vi "Set Object ACL.vi"(6 "Version ID":string, 8 "error in (no error)":errorcluster, 9 "Access Control Policy":T1, 10 "Object Path":string, 11 "Bucket in":refnum<class "Bucket.lvclass">) -> (0 "error out":errorcluster, 3 "Bucket out":refnum<class "Bucket.lvclass">)   [LabVIEW 2015, in "NI_AWS_S3.lvlib" / "Bucket.lvclass"]
uses:
  Bucket.lvclass
  Access Control Policy.ctl
  User.ctl
  Grantee-Permission Pair.ctl
  Permission.ctl
  Core/HTTP Request/Request Options.ctl
  Core/HTTP Request/Name Value Pair.ctl
  Core/HTTP Request/Region handling.ctl
  Core/HTTP Request/URL formatting.ctl
  Bucket.lvclass/Bucket.ctl
  Read Name.vi
  Core/HTTP Request/HTTP Request.lvclass
  NI_AWS_S3.lvlib
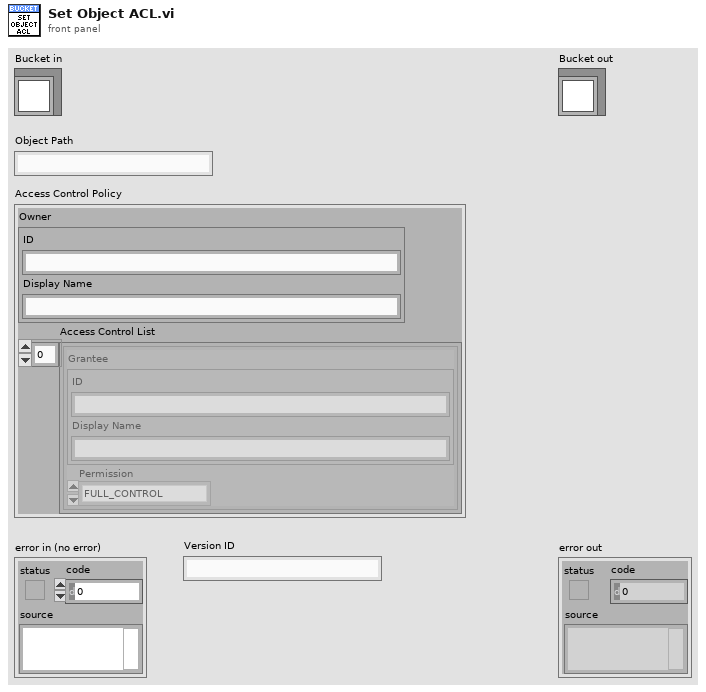
[diagram p1: front panel]
types:
  T1 = typedef "NI_AWS_S3.lvlib/Access Control Policy.ctl" = cluster{"Owner":T2, "Access Control List":T3[]}
  T2 = typedef "NI_AWS_S3.lvlib/User.ctl" = cluster{"ID":string, "Display Name":string}
  T3 = typedef "NI_AWS_S3.lvlib/Grantee-Permission Pair.ctl" = cluster{"Grantee":T2, "Permission":T4}
  T4 = typedef "NI_AWS_S3.lvlib/Permission.ctl" = enum16{"FULL_CONTROL", "WRITE", "WRITE_ACP", "READ", "READ_ACP"}
  T5 = typedef "NI_AWS_Core.lvlib/HTTP Request.lvclass/Name Value Pair.ctl" = cluster{"name":string, "value":string}
  T6 = typedef "NI_AWS_Core.lvlib/HTTP Request.lvclass/Region handling.ctl" = enum16{"use region everywhere", "use region (authentication only)", "use region (URL only)", "ignore region everwhere"}
  T7 = typedef "NI_AWS_Core.lvlib/HTTP Request.lvclass/Request Options.ctl" = cluster{"request headers":T5[], "request parameters":T5[], "request body":string, "region handling":T6, "URL formatting":T8}
  T8 = typedef "NI_AWS_Core.lvlib/HTTP Request.lvclass/URL formatting.ctl" = enum16{"region-", "region."}
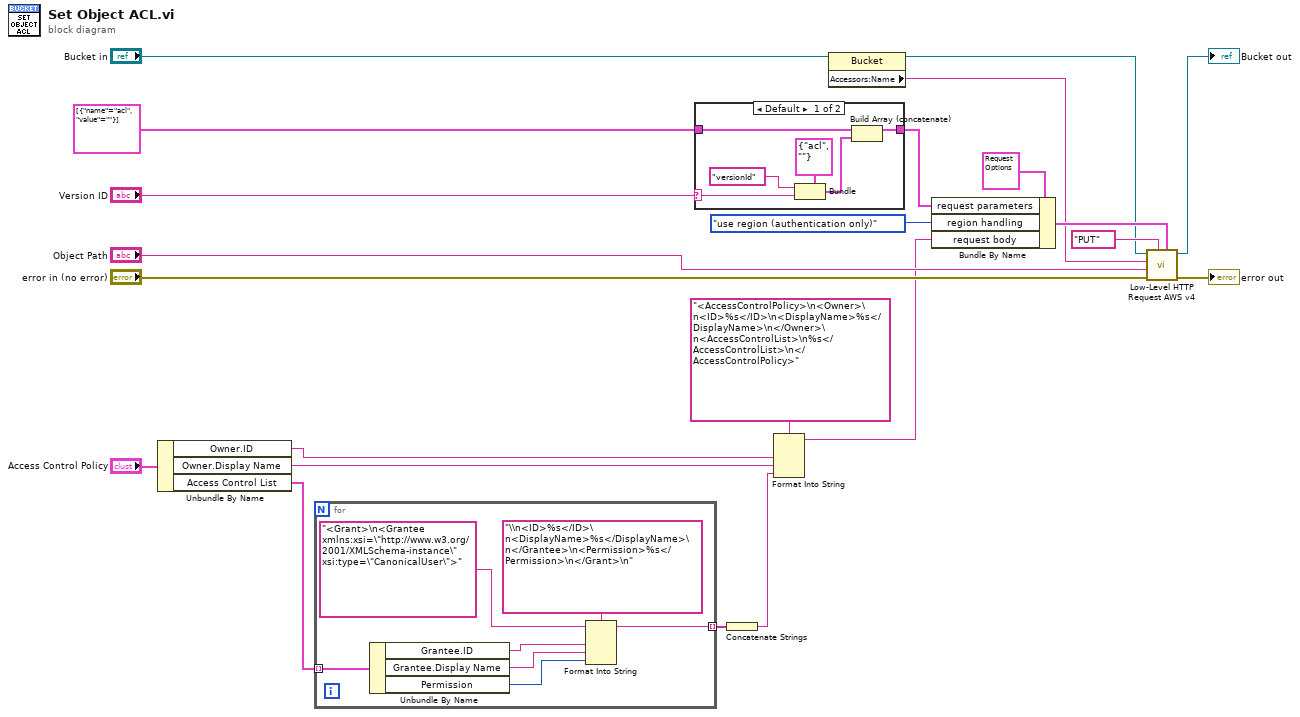
[diagram p0: block diagram]
diagram:
  n1 = Unbundle By Name("Access Control Policy") -> ("Owner.ID"=w5:string, "Owner.Display Name"=w6:string, "Access Control List"=w4:T3[])
  n2 = for {
    tunnel: w4 -> [w29] mode=indexing
    tunnel: [w23] -> w3 mode=indexing
    n3 = Unbundle By Name(w29) -> ("Grantee.ID"=w26:string, "Grantee.Display Name"=w25:string, "Permission"=w24:T4)
    n4 = Format Into String(format string="\\n<ID>%s</ID>\n<DisplayName>%s</DisplayName>\n</Grantee>\n<Permission>%s</Permission>\n</Grant>\n", initial string="<Grant>\n<Grantee xmlns:xsi=\"http://www.w3.org/2001/XMLSchema-instance\" xsi:type=\"CanonicalUser\">", w26, w25, w24) -> (resulting string=w23:string)  [unwired: 1 in, 1 out]
  }
  n5 = case shown="Default" "Version ID" {
    selector: "Version ID" -> [w32 _]
    tunnel: [w33 w36] -> w18
    tunnel: T5[] [{"name"="acl", "value"=""}] ("appended array") -> [w31 w36]
    frame Default {
      n6 = Bundle(cluster=T5 {"name"="acl", "value"=""}, "name"="versionId", "value"=w32) -> (w34:T5)
      n7 = Build Array (concatenate)(w31, w34) -> (w33:T5[])
    }
    frame "" {
    }
  }
  n8 = Concatenate Strings(w3) -> (w2:string)
  n9 = Format Into String(format string="<AccessControlPolicy>\n<Owner>\n<ID>%s</ID>\n<DisplayName>%s</DisplayName>\n</Owner>\n<AccessControlList>\n%s</AccessControlList>\n</AccessControlPolicy>", w5, w6, w2) -> (resulting string=w8:string)  [unwired: 2 in, 1 out]
  n10 = property class="Bucket"(reference="Bucket in") -> (reference out=w14:refnum<class "Bucket.lvclass">, "Accessors:Name"=w13:string)  [unwired: 1 in, 1 out]
  n11 = Bundle By Name(cluster=T7 {"request headers"=[], "request parameters"=[], "request body"="", "region handling"=enum."use region everywhere", "URL formatting"=enum."region."} ("Request Options"), "request parameters"=w18, "region handling"=Region_handling."use region (authentication only)", "request body"=w8) -> (w19:T7)
  n12 = call "Low-Level HTTP Request AWS v4.vi"("Request Options"=w19, "HTTP-Verb"="PUT", "error in (no error)"="error in (no error)", "URL Suffix"="Object Path", "URL Prefix"=w13, "AWS Core in"=w14) -> ("error out"=→"error out":errorcluster, "AWS Core out"=→"Bucket out":refnum<class "Bucket.lvclass">)  [unwired: 2 in, 2 out]
